vi "VI 서버 설명.vi"() -> ()   [LabVIEW 2014]
panel:
  in  "vi 경로":path
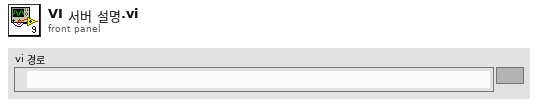
[diagram p1: front panel]
types:
  T1 = enum8{"Enabled", "Disabled", "Disabled and Grayed Out"}
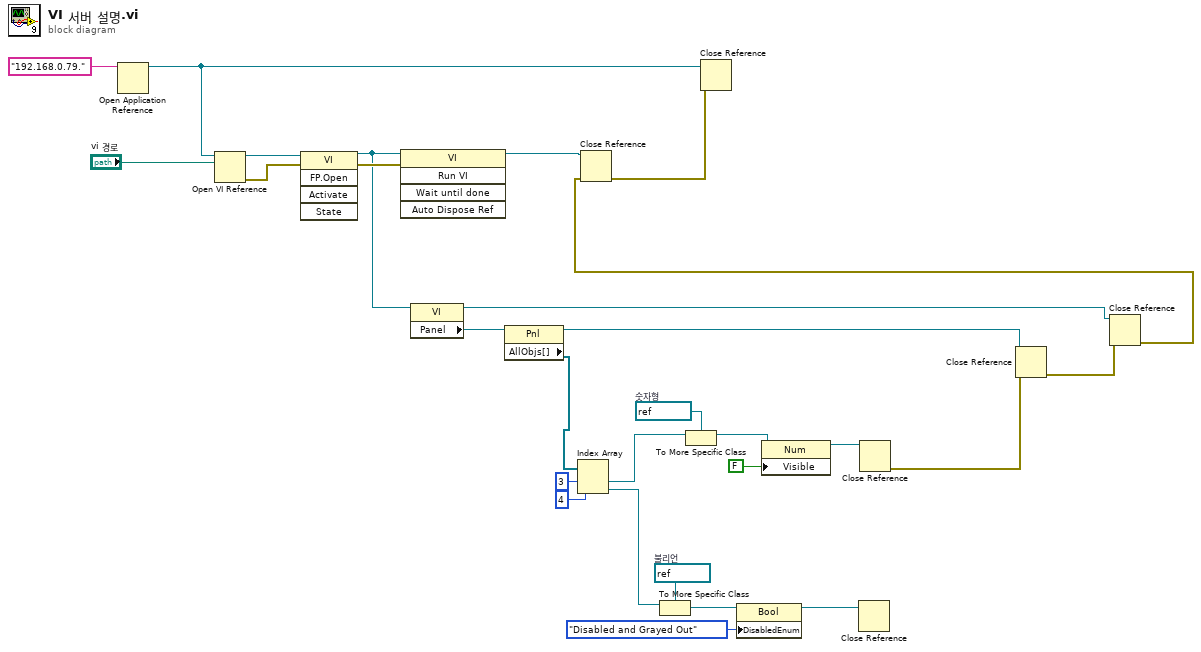
[diagram p0: block diagram]
diagram:
  w20 = refnum<vi> refnum  # 숫자형
  w21 = refnum<vi> refnum  # 불리언
  n1 = Open Application Reference(11:"192.168.0.79." ("머신 이름(\"\":  로컬 참조 열기)")) -> (3:w9:refnum<vi>)  [unwired: 3 in, 1 out]
  n2 = Open VI Reference(application reference (local)=w9, vi path="vi 경로") -> (vi reference=w27:refnum<vi>, error out=w26:errorcluster)  [unwired: 4 in]
  n3 = invoke class="VI" method="FP.Open"(reference=w27, error in=w26) -> (reference out=w23:refnum<vi>, error out=w25:errorcluster)  [unwired: 3 in, 3 out]
  n4 = invoke class="VI" method="Run VI"(reference=w23, error in=w25) -> (reference out=w24:refnum<vi>)  [unwired: 3 in, 4 out]
  n5 = property class="VI"(reference=w23) -> (reference out=w3:refnum<vi>, "Panel"=w22:refnum<vi>)  [unwired: 1 in, 1 out]
  n6 = property class="Pnl"(reference=w22) -> (reference out=w5:refnum<vi>, "AllObjs[]"=w11:refnum<vi>[])  [unwired: 1 in, 1 out]
  n7 = Index Array(array=w11, index #1=3 ("인덱스"), index #2=4 ("인덱스")) -> (element #1=w15:refnum<vi>, element #2=w14:refnum<vi>)
  n8 = To More Specific Class(target class=w21, reference=w14) -> (specific class reference=w19:refnum<vi>)  [unwired: 1 in, 1 out]
  n9 = To More Specific Class(target class=w20, reference=w15) -> (specific class reference=w18:refnum<vi>)  [unwired: 1 in, 1 out]
  n10 = property class="Bool"(reference=w19, "DisabledEnum"=T1."Disabled and Grayed Out" ("비활성화")) -> (reference out=w6:refnum<vi>)  [unwired: 1 in, 1 out]
  n11 = property class="Num"(reference=w18, "Visible"=FALSE ("보이기")) -> (reference out=w7:refnum<vi>)  [unwired: 1 in, 1 out]
  n12 = Close Reference(reference=w6) -> ()  [unwired: 1 in, 1 out]
  n13 = Close Reference(reference=w7) -> (error out=w4:errorcluster)  [unwired: 1 in]
  n14 = Close Reference(reference=w5, error in (no error)=w4) -> (error out=w2:errorcluster)
  n15 = Close Reference(reference=w3, error in (no error)=w2) -> (error out=w1:errorcluster)
  n16 = Close Reference(reference=w24, error in (no error)=w1) -> (error out=w8:errorcluster)
  n17 = Close Reference(reference=w9, error in (no error)=w8) -> ()  [unwired: 1 out]
